vi "Run Bfr Tx - Handle Transmit Size.vi"(8 "error in (no error)":errorcluster, 11 "Transmit Bytes":T1) -> (0 "error out":errorcluster, 2 "Bytes to Transmit":i32, 3 "Transmit?":bool)   [LabVIEW 2016, in "UDP-Custom-Device Engine.lvlib"]
uses:
  UDP-Custom-Device Engine.lvlib
  <vilib>/NI/NIVS Inline Async API/_Data Access Engine/Data Access Engine/Types/Read.DVR.ctl
  <vilib>/NI/NIVS Inline Async API/_Data Access Engine/Access Type Classes/Read/Read.lvclass
  <vilib>/NI/NIVS Inline Async API/_Data Access Engine/Access Type Classes/Read/Read.lvclass/Read.ctl
  <vilib>/NI Veristand/VeriStand Data/Library/Type Conversion/Type Conversion.From Double (I32).vi
  <vilib>/NI/NIVS Inline Async API/_Data Access Engine/Data Access Engine/Methods/Read.Data.vi
  <vilib>/NI/NIVS Inline Async API/_Data Access Engine/Access Type Classes/Read/Read.ProcessData.vi
  <vilib>/NI Veristand/VeriStand Data/Library/VeriStand Data.lvlib
  <vilib>/NI/NIVS Inline Async API/_Data Access Engine/Data Access Engine/Data Access Engine.lvclass
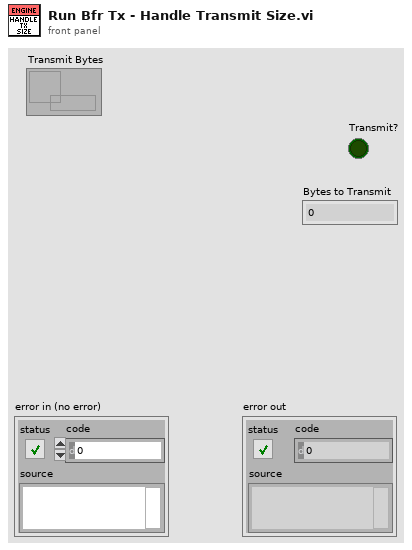
[diagram p1: front panel]
types:
  T1 = typedef "Data Access Engine.lvlib/Data Access Engine.lvclass/Read.DVR.ctl" = refnum<data-value>
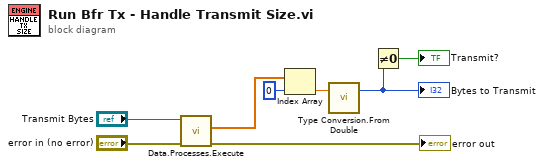
[diagram p0: block diagram]
diagram:
  n1 = call-poly <vilib>:"Data.Processes.Execute.vi"("error in (no error)"="error in (no error)", "Ref"="Transmit Bytes") -> ("error out"=→"error out":errorcluster, "Values"=w8:dbl[])  [unwired: 7 in, 1 out]
  n2 = Index Array(array=w8, index=0) -> (element=w6:dbl)
  n3 = call-poly <vilib>:"Type Conversion.From Double.vi"("value in"=w6) -> ("value out"=w2:i32)  [unwired: 2 in]
  "Bytes to Transmit" <- w2
  n4 = Not Equal To 0?(x=w2) -> (x != 0?=→"Transmit?":bool)
